vi "TRIG_config_UI.vi"() -> ()   [LabVIEW 2011]
uses:
  global.vi
  <vilib>/Platform/browser.llb/Open URL in Default Browser (string).vi
panel:
  in  "Close":bool
  in  "BG cycle":dbl=100.0 min=0.0 max=999.999999999995 format="%.2f"
  in  "mol. delay":dbl=100.0 min=0.0 max=999.999999999995 format="%.2f"
  in  "Reset TRIG":bool
  in  "write config":bool
  out "Burst enable":bool=TRUE caption="Burst"
  out "Digital Waveform Graph":digitalwaveform(graph)={"t0"=timestamp(0 s since 1904-01-01), "dt"=3e-08, "Y"={"transitions"=[], "data"=array4950x4[19800 elements]}}
  in  "burst period":dbl=49.99999999999998 min=1e-07 format="%.2f"
  in  "burst count":i32=3 min=1
  in  "duration":dbl[](array[numeric])=[5.65, 5.0, 40.0, 5.0] min=0.0 format="%.3f"
  in  "start time":dbl[](array[numeric])=[0.0, 1.1, 6.6000000000000005, 6.3999999999999995] format="%.3f"
  in  "time unit":enum16{"s", "ms", "us", "ns"}(ring)=enum."us"
  in  "help":bool
  out "update front panel":bool
  # "Configure Delay Generator (TRIG)"
  # "power AMP"
  # "AWG"
  # "SWITCH"
  # "OSC"
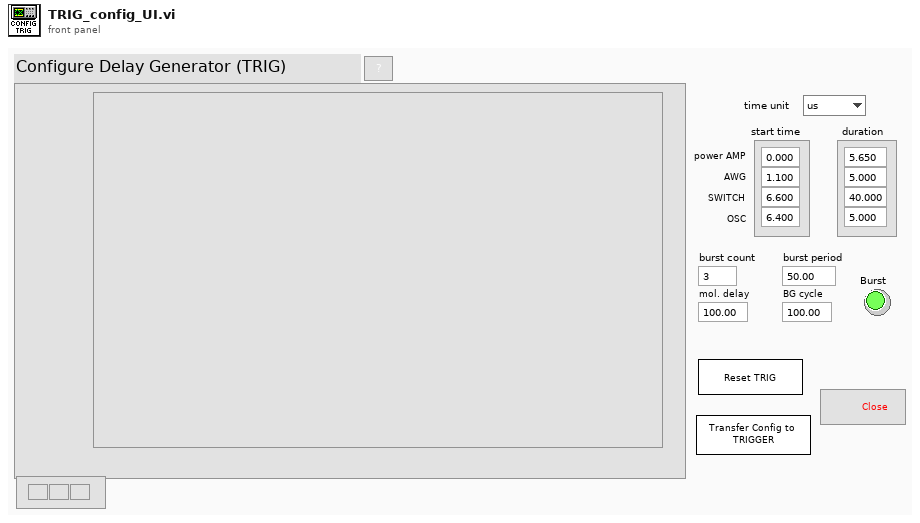
[diagram p1: front panel]
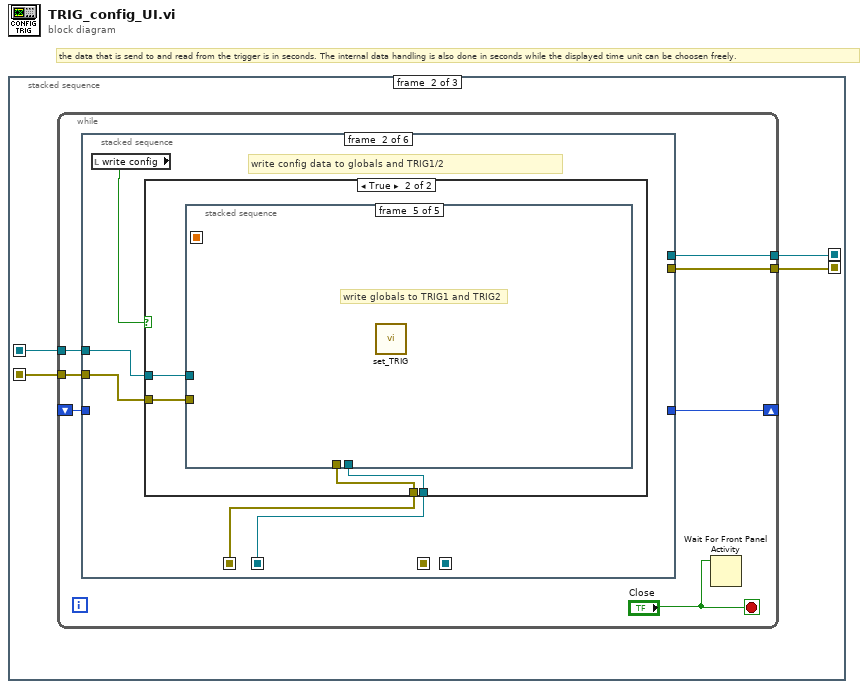
[diagram p0: block diagram]
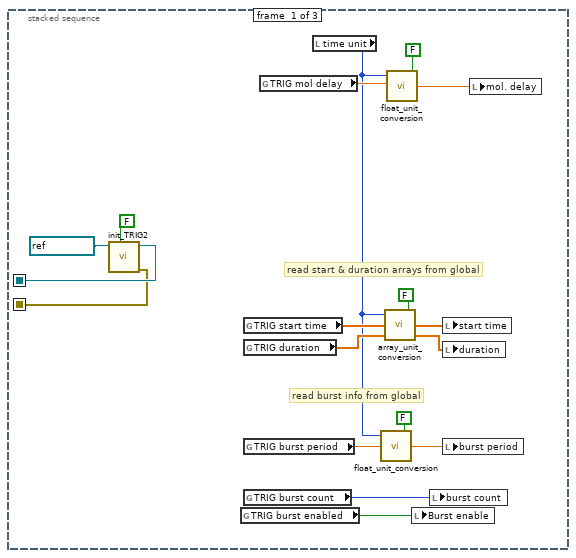
[diagram p2: hidden frame]
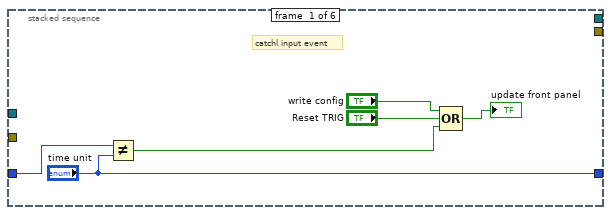
[diagram p3: hidden frame]
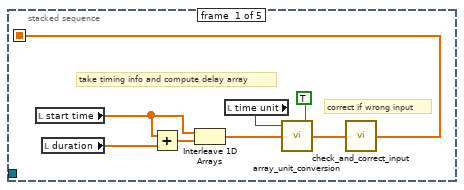
[diagram p5: hidden frame]
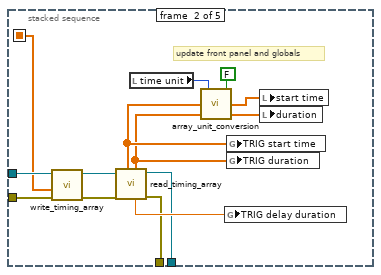
[diagram p6: hidden frame]
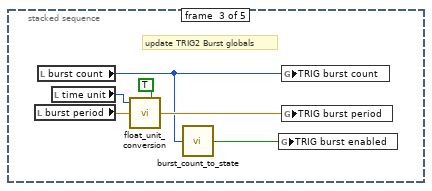
[diagram p7: hidden frame]
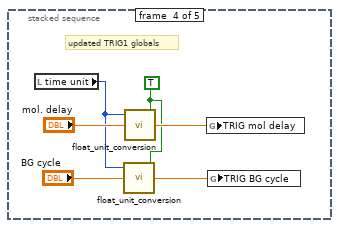
[diagram p8: hidden frame]
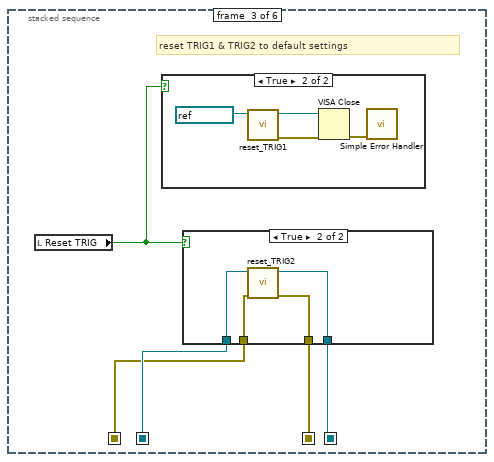
[diagram p9: hidden frame]
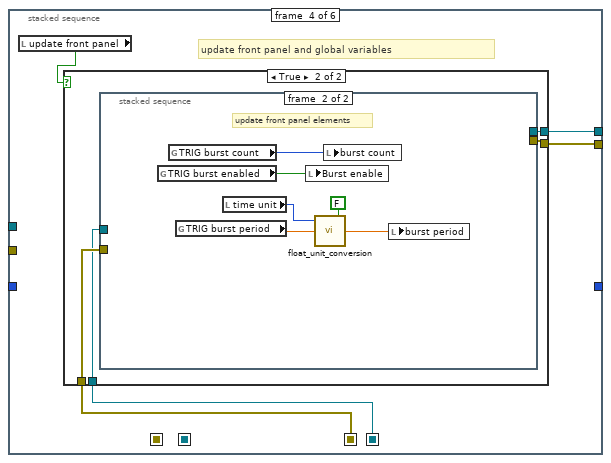
[diagram p12: hidden frame]
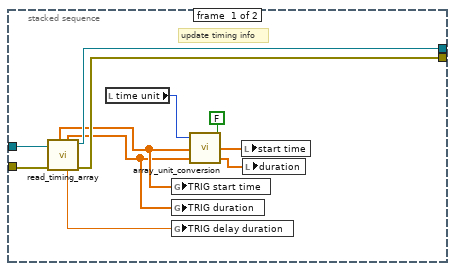
[diagram p14: hidden frame]
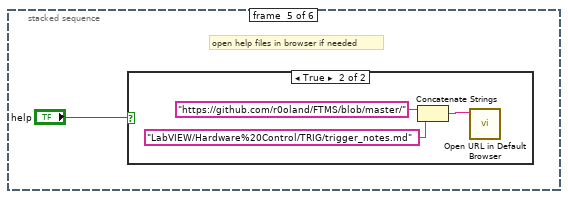
[diagram p15: hidden frame]
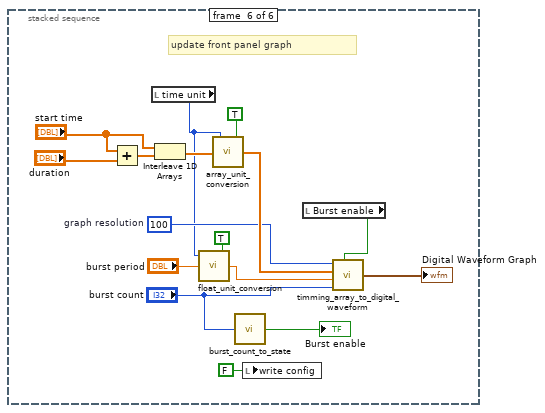
[diagram p17: hidden frame]
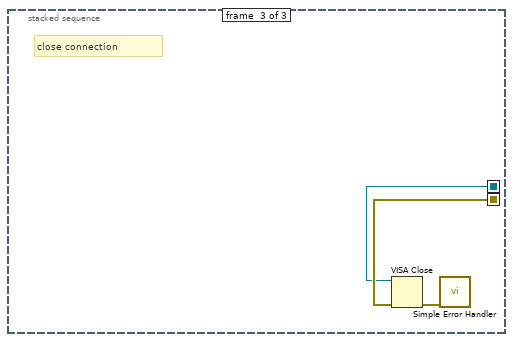
[diagram p18: hidden frame]
diagram:
  # "the data that is send to and read from the trigger is in seconds. The internal data handling is also done in seconds while the displayed time unit can be choosen freely."
  n1 = stacked-sequence {
    seq-local: [w15 _ _] -> [_ w22 _]
    seq-local: [w14 _ _] -> [_ w21 _]
    seq-local: [_ w20 _] -> [_ _ w144]
    seq-local: [_ w19 _] -> [_ _ w146]
    frame #0 {
      # "read burst info from global"
      # "read start & duration arrays from global"
      n2 = call "init_TRIG2.vi"("reset TRIG"=FALSE, "VISA resource name"=refnum<visa-resource-name> "TRIG2" ("TRIG2 resource name")) -> ("error out"=w14:errorcluster, "VISA resource name out"=w15:refnum<visa-resource-name>)  [unwired: 5 in]
      n3 = global read "global.vi" "TRIG burst enabled"() -> (w1:bool)
      n4 = global read "global.vi" "TRIG start time"() -> (w13:dbl[])
      n5 = global read "global.vi" "TRIG duration"() -> (w11:dbl[])
      n6 = global read "global.vi" "TRIG burst period"() -> (w6:dbl)
      n7 = global read "global.vi" "TRIG burst count"() -> (w9:i32)
      n8 = global read "global.vi" "TRIG mol delay"() -> (w4:dbl)
      n9 = local read "time unit"() -> (w3:enum16{"s", "ms", "us", "ns"})
      n10 = call "float_unit_conversion.vi"("inverse function (arb. unit to s)?"=FALSE, "time"=w6, "time unit"=w3) -> ("converted time"=w7:dbl)  [unwired: 2 in]
      n11 = call "array_unit_conversion.vi"("inverse function (arb. unit to s)?"=FALSE, "delay array 2"=w11, "delay array"=w13, "time unit"=w3) -> ("output 2"=w10:dbl[], "output"=w12:dbl[])
      n12 = call "float_unit_conversion.vi"("inverse function (arb. unit to s)?"=FALSE ("inverse"), "time"=w4, "time unit"=w3) -> ("converted time"=w2:dbl)  [unwired: 2 in]
      n13 = local write "Burst enable"(w1) -> ()
      n14 = local write "burst count"(w9) -> ()
      n15 = local write "start time"(w12) -> ()
      n16 = local write "duration"(w10) -> ()
      n17 = local write "burst period"(w7) -> ()
      n18 = local write "mol. delay"(w2) -> ()
    }
    frame #1 {
      n19 = while {
        tunnel: w21 -> [w27]
        tunnel: [w29] -> w20
        tunnel: [w28] -> w19
        tunnel: w22 -> [w26]
        shift-right: [w25] -> _
        shift-left: _ -> [w24]
        stop <- "Close" stop-if-true
        n20 = stacked-sequence {
          seq-local: [_ w36 _ _ _ _] -> [_ _ w81 _ _ _]
          seq-local: [_ w37 _ _ _ _] -> [_ _ w82 _ _ _]
          seq-local: [_ _ w84 _ _ _] -> [_ _ _ w99 _ _]
          seq-local: [_ _ w85 _ _ _] -> [_ _ _ w98 _ _]
          tunnel: w26 -> [_ w39 _ _ _ _]
          tunnel: w27 -> [_ w38 _ _ _ _]
          tunnel: [_ _ _ w97 _ _] -> w28
          tunnel: [_ _ _ w100 _ _] -> w29
          tunnel: ["time unit" _ _ _ _ _] -> w25
          tunnel: w24 -> [w32 _ _ _ _ _]
          frame #0 {
            # "catchl input event"
            n21 = Not Equal?(x=w32, y="time unit") -> (x != y?=w33:bool)
            n22 = Compound Arithmetic op=OR("write config", "Reset TRIG", w33) -> (→"update front panel":bool)
          }
          frame #1 {
            # "write config data to globals and TRIG1/2"
            n23 = local read "write config"() -> (w40:bool)
            n24 = case shown="True" w40 {
              tunnel: w39 -> [w42 w46]
              tunnel: w38 -> [w41 w45]
              tunnel: [w42 w44] -> w37
              tunnel: [w41 w43] -> w36
              frame False {
              }
              frame True {
                n25 = stacked-sequence {
                  seq-local: [w47 _ _ _ _] -> [_ w57 _ _ _]
                  tunnel: w46 -> [_ w61 _ _ _]
                  tunnel: w45 -> [_ w60 _ _ _]
                  tunnel: [_ w56 _ _ _] -> w44
                  tunnel: [_ w55 _ _ _] -> w43
                  frame #0 {
                    # "correct if wrong input"
                    # "take timing info and compute delay array"
                    n26 = local read "start time"() -> (w49:dbl[])
                    n27 = local read "duration"() -> (w48:dbl[])
                    n28 = Add(x=w49, y=w48) -> (x+y=w53:dbl[])
                    n29 = Interleave 1D Arrays(w49, w53) -> (w51:dbl[])
                    n30 = local read "time unit"() -> (w50:enum16{"s", "ms", "us", "ns"})
                    n31 = call "array_unit_conversion.vi"("inverse function (arb. unit to s)?"=TRUE, "delay array"=w51, "time unit"=w50) -> ("output"=w54:dbl[])  [unwired: 1 in, 1 out]
                    n32 = call "check_and_correct_input.vi"("delay array"=w54) -> ("corrrected delay array"=w47:dbl[])  [unwired: 4 in]
                  }
                  frame #1 {
                    # "update front panel and globals"
                    n33 = call "write_timing_array.vi"("error in"=w60, "delay array"=w57, "VISA resource in"=w61) -> ("error out 2"=w58:errorcluster, "VISA resource out"=w59:refnum<visa-resource-name>)  [unwired: 3 in]
                    n34 = call "read_timing_array.vi"("error in"=w58, "VISA resource in"=w59) -> ("error out 2"=w55:errorcluster, "VISA resource out"=w56:refnum<visa-resource-name>, "delay duration"=w64:dbl, "duration"=w62:dbl[], "start time"=w63:dbl[])  [unwired: 5 in]
                    n35 = local read "time unit"() -> (w67:enum16{"s", "ms", "us", "ns"})
                    n36 = call "array_unit_conversion.vi"("inverse function (arb. unit to s)?"=FALSE, "delay array 2"=w62, "delay array"=w63, "time unit"=w67) -> ("output 2"=w65:dbl[], "output"=w66:dbl[])
                    n37 = global write "global.vi" "TRIG delay duration"(w64) -> ()
                    n38 = global write "global.vi" "TRIG start time"(w63) -> ()
                    n39 = global write "global.vi" "TRIG duration"(w62) -> ()
                    n40 = local write "start time"(w66) -> ()
                    n41 = local write "duration"(w65) -> ()
                  }
                  frame #2 {
                    # "update TRIG2 Burst globals"
                    n42 = local read "burst period"() -> (w74:dbl)
                    n43 = local read "burst count"() -> (w69:i32)
                    n44 = local read "time unit"() -> (w72:enum16{"s", "ms", "us", "ns"})
                    n45 = call "float_unit_conversion.vi"("inverse function (arb. unit to s)?"=TRUE, "time"=w74, "time unit"=w72) -> ("converted time"=w71:dbl)  [unwired: 2 in]
                    n46 = call "burst_count_to_state.vi"("burst count"=w69) -> ("Burst On"=w70:bool)  [unwired: 4 in]
                    n47 = global write "global.vi" "TRIG burst enabled"(w70) -> ()
                    n48 = global write "global.vi" "TRIG burst count"(w69) -> ()
                    n49 = global write "global.vi" "TRIG burst period"(w71) -> ()
                  }
                  frame #3 {
                    w76 = TRUE ("inverse")
                    # "updated TRIG1 globals"
                    n50 = local read "time unit"() -> (w77:enum16{"s", "ms", "us", "ns"})
                    n51 = call "float_unit_conversion.vi"("inverse function (arb. unit to s)?"=w76, "time"="BG cycle", "time unit"=w77) -> ("converted time"=w75:dbl)  [unwired: 2 in]
                    n52 = call "float_unit_conversion.vi"("inverse function (arb. unit to s)?"=w76, "time"="mol. delay", "time unit"=w77) -> ("converted time"=w79:dbl)  [unwired: 2 in]
                    n53 = global write "global.vi" "TRIG mol delay"(w79) -> ()
                    n54 = global write "global.vi" "TRIG BG cycle"(w75) -> ()
                  }
                  frame #4 {
                    # "write globals to TRIG1 and TRIG2"
                    n55 = call "set_TRIG.vi"() -> ()  [unwired: 12 in]
                  }
                }
              }
            }
          }
          frame #2 {
            # "reset TRIG1 & TRIG2 to default settings"
            n56 = local read "Reset TRIG"() -> (w83:bool)
            n57 = case shown="True" w83 {
              frame False {
              }
              frame True {
                n58 = call "reset_TRIG1.vi"("VISA resource name"=refnum<visa-resource-name> "TRIG1") -> ("error out"=w86:errorcluster, "VISA resource name out"=w87:refnum<visa-resource-name>)  [unwired: 9 in]
                n59 = VISA Close(VISA resource name=w87, error in (no error)=w86) -> (error out=w88:errorcluster)
                n60 = call <vilib>:"Simple Error Handler.vi"("error in (no error)"=w88) -> ()  [unwired: 4 in, 5 out]
              }
            }
            n61 = case shown="True" w83 {
              tunnel: w81 -> [w90 w92]
              tunnel: w82 -> [w91 w93]
              tunnel: [w91 w94] -> w85
              tunnel: [w90 w95] -> w84
              frame False {
              }
              frame True {
                n62 = call "reset_TRIG2.vi"("error in (no error)"=w92, "VISA resource name"=w93) -> ("error out"=w95:errorcluster, "VISA resource name out"=w94:refnum<visa-resource-name>)  [unwired: 8 in]
              }
            }
          }
          frame #3 {
            # "update front panel and global variables"
            n63 = local read "update front panel"() -> (w96:bool)
            n64 = case shown="True" w96 {
              tunnel: [w102 w106] -> w100
              tunnel: [w101 w105] -> w97
              tunnel: w99 -> [w101 w104]
              tunnel: w98 -> [w102 w103]
              frame False {
              }
              frame True {
                n65 = stacked-sequence {
                  tunnel: [w117 _] -> w106
                  tunnel: [w116 _] -> w105
                  tunnel: w104 -> [w115 _]
                  tunnel: w103 -> [w114 _]
                  frame #0 {
                    # "update timing info"
                    n66 = call "read_timing_array.vi"("error in"=w115, "VISA resource in"=w114) -> ("error out 2"=w116:errorcluster, "VISA resource out"=w117:refnum<visa-resource-name>, "delay duration"=w108:dbl, "duration"=w109:dbl[], "start time"=w110:dbl[])  [unwired: 5 in]
                    n67 = local read "time unit"() -> (w107:enum16{"s", "ms", "us", "ns"})
                    n68 = global write "global.vi" "TRIG start time"(w110) -> ()
                    n69 = global write "global.vi" "TRIG duration"(w109) -> ()
                    n70 = global write "global.vi" "TRIG delay duration"(w108) -> ()
                    n71 = call "array_unit_conversion.vi"("inverse function (arb. unit to s)?"=FALSE, "delay array 2"=w109, "delay array"=w110, "time unit"=w107) -> ("output 2"=w111:dbl[], "output"=w112:dbl[])
                    n72 = local write "start time"(w112) -> ()
                    n73 = local write "duration"(w111) -> ()
                  }
                  frame #1 {
                    # "update front panel elements"
                    n74 = global read "global.vi" "TRIG burst enabled"() -> (w118:bool)
                    n75 = global read "global.vi" "TRIG burst count"() -> (w123:i32)
                    n76 = global read "global.vi" "TRIG burst period"() -> (w121:dbl)
                    n77 = local read "time unit"() -> (w120:enum16{"s", "ms", "us", "ns"})
                    n78 = local write "Burst enable"(w118) -> ()
                    n79 = call "float_unit_conversion.vi"("inverse function (arb. unit to s)?"=FALSE, "time"=w121, "time unit"=w120) -> ("converted time"=w119:dbl)  [unwired: 2 in]
                    n80 = local write "burst count"(w123) -> ()
                    n81 = local write "burst period"(w119) -> ()
                  }
                }
              }
            }
          }
          frame #4 {
            # "open help files in browser if needed"
            n82 = case shown="True" "help" {
              frame False {
              }
              frame True {
                n83 = Concatenate Strings("https://github.com/r0oland/FTMS/blob/master/" ("string"), "LabVIEW/Hardware%20Control/TRIG/trigger_notes.md" ("string")) -> (w127:string)
                n84 = call-poly <vilib>:"Open URL in Default Browser.vi"("URL"=w127) -> ()  [unwired: 5 in, 2 out]
              }
            }
          }
          frame #5 {
            w139 = 100  # graph resolution
            # "update front panel graph"
            n85 = Add(x="start time", y="duration") -> (x+y=w143:dbl[])
            n86 = local read "time unit"() -> (w133:enum16{"s", "ms", "us", "ns"})
            n87 = Interleave 1D Arrays("start time", w143) -> (w141:dbl[])
            n88 = call "float_unit_conversion.vi"("inverse function (arb. unit to s)?"=TRUE, "time"="burst period", "time unit"=w133) -> ("converted time"=w132:dbl)  [unwired: 2 in]
            n89 = call "array_unit_conversion.vi"("inverse function (arb. unit to s)?"=TRUE, "delay array"=w141, "time unit"=w133) -> ("output"=w140:dbl[])  [unwired: 1 in, 1 out]
            n90 = call "burst_count_to_state.vi"("burst count"="burst count") -> ("Burst On"=→"Burst enable":bool)  [unwired: 4 in]
            n91 = local write "write config"(FALSE ("write config")) -> ()
            n92 = local read "Burst enable"() -> (w130:bool)
            n93 = call "timming_array_to_digital_waveform.vi"("resolution"=w139, "delay array"=w140, "burst period"=w132, "burst count"="burst count", "Burst?"=w130) -> ("digital waveform"=→"Digital Waveform Graph":digitalwaveform)  [unwired: 2 in]
          }
        }
        n94 = Wait For Front Panel Activity(3:"Close") -> ()  [unwired: 2 in, 1 out]
      }
    }
    frame #2 {
      # "close connection"
      n95 = VISA Close(VISA resource name=w144, error in (no error)=w146) -> (error out=w145:errorcluster)
      n96 = call <vilib>:"Simple Error Handler.vi"("error in (no error)"=w145) -> ()  [unwired: 4 in, 5 out]
    }
  }
